vi "add_string_roslv.vi"   [LabVIEW 2014]
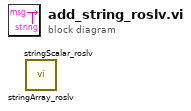
[diagram p0: block diagram]
diagram:
  n1 = call "stringArray_roslv.vi"() -> ()  [unwired: 5 in, 1 out]
  n2 = call "stringScalar_roslv.vi"() -> ()  [unwired: 5 in, 1 out]
